vi "流程文件XML解析.vi"(10 "添加的路径":path, 11 "参数簇":cluster{"启动参数":u16, "启动模式":u16, "量程":u16}={"启动参数"=1, "启动模式"=0, "量程"=0} {"量程" items=["低量程", "高量程"]; "启动参数" items=["CODMn"=21, "总磷"=1, "总氮"=2, "氨氮"=3]; "启动模式" items=["", "水样测量", "标样核查", "零点核查", "跨度核查", "空白测试", "平行样测试", "加标回收", "填充管路", "清洗管路", "清洗反应杯"]}) -> (3 "数组":T1(array[cluster]))   [LabVIEW 2016, in "挥发酚.lvlib"]
uses:
  <vilib>/xml/Load XML File.vi
  <vilib>/xml/Close Reference(Node).vi
  <resource>/objmgr/DOMUserDefRef.rc
  <vilib>/xml/NI_XML.lvlib
panel:
  out "大小":i32
  out "XML字符串":string="<?xml version=\"1.0\" encoding=\"ISO-8859-1\"?>\n<bookstore>\n<book ISBN=\"978-0545128285\">\n  <title lang=\"en\">The Tales of Beedle the Bard</title>\n  <author>J. K. Rowling</author>\n  <year>2008</year>\n  <price>12.99</price>\n</book>\n<book ISBN=\"978-0316160209\">\n  <title lang=\"en\">Eclipse</title>\n  <author>Stephenie Meyer</author>\n  <year>2007</year>\n  <price>19.99</price>\n</book>\n<book ISBN=\"978-0316067928\">\n  <title lang=\"en\">Breaking Dawn</title>\n  <author>Stephenie Meyer</author>\n  <year>2008</year>\n  <price>22.99</price>\n</book>\n<book ISBN=\"978-0316017923\">\n  <title lang=\"en\">Outliers: The Story of Success</title>\n  <author>Malcolm Gladwell</author>\n  <year>2008</year>\n  <price>27.99</price>\n</book>\n<book ISBN=\"978-0596007645\">\n  <title lang=\"en\">XML in a Nutshell</title>\n  <author>Elliotte Rusty Harold</author>\n  <author>W. Scott Means</author>\n  <year>2004</year>\n  <price>39.95</price>\n</book>\n</bookstore>"
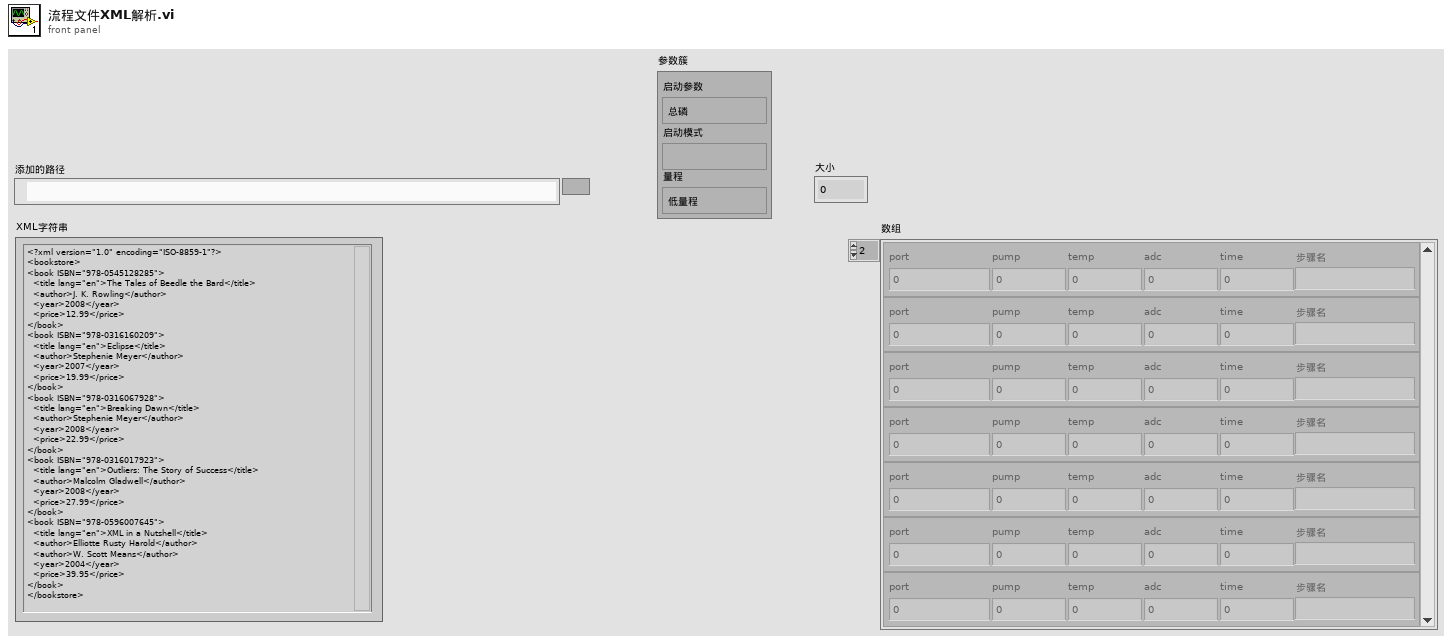
[diagram p1: front panel]
types:
  T1 = cluster{"port":u32, "pump":u16, "temp":u8, "adc":u8, "time":u16, "步骤名":string}[]
  T2 = cluster{"port":u32, "pump":u16, "temp":u8, "adc":u8, "time":u16, "步骤名":string}
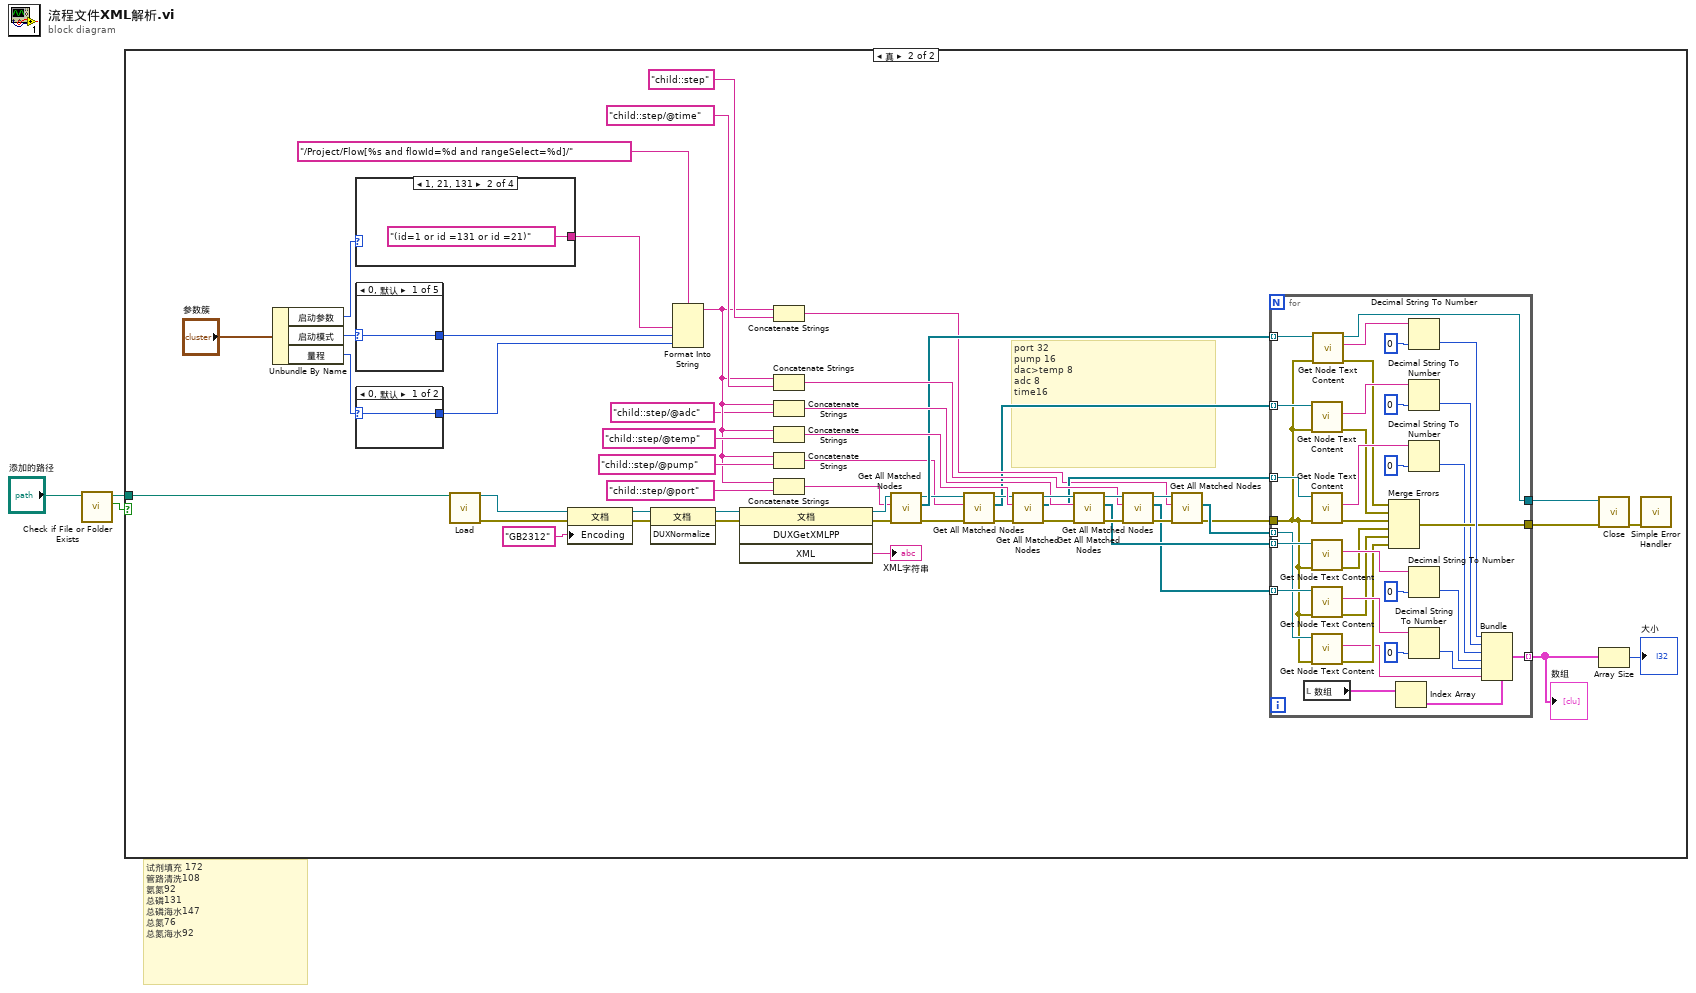
[diagram p0: block diagram]
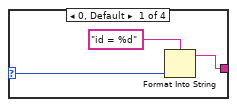
[diagram p3: hidden frame]
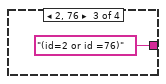
[diagram p4: hidden frame]
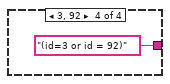
[diagram p5: hidden frame]
diagram:
  # "试剂填充 172 \n管路清洗108\n氨氮92\n总磷131\n总磷海水147\n总氮76\n总氮海水92"
  n1 = call <vilib>:"Check if File or Folder Exists.vi"("path"="添加的路径") -> ("file or folder exists?"=w1:bool, "dup path"=w2:path)  [unwired: 8 in, 1 out]
  n2 = case shown="真" w1 {
    tunnel: w2 -> [_ w40]
    frame False {
    }
    frame True {
      # "port 32\npump 16\ndac>temp 8\nadc 8\ntime16"
      n3 = Unbundle By Name("参数簇") -> ("启动参数"=w42:u16, "启动模式"=w45:u16, "量程"=w44:u16)
      n4 = case shown="1, 21, 131" w42 {
        selector: w42 -> [w93 _ _ _]
        tunnel: [w92 "(id=1 or id =131 or id =21)" ("输入 4") "(id=2 or id =76)" ("输入 4") "(id=3 or id = 92)" ("输入 4")] -> w41
        frame 0, Default {
          n5 = Format Into String(format string="id = %d" ("格式字符串"), w93) -> (resulting string=w92:string)  [unwired: 2 in, 1 out]
        }
        frame 1, 21, 131 {
        }
        frame 2, 76 {
        }
        frame 3, 92 {
        }
      }
      n6 = case shown="0, 默认" w45 {
        selector: w45 -> [w100 w101 w102 w103 w104]
        tunnel: [w100 w101 w102 w103 w104] -> w48
        frame 0, Default {
        }
        frame 1 {
        }
        frame 2 {
        }
        frame 3 {
        }
        frame 4 {
        }
      }
      n7 = case shown="0, 默认" w44 {
        selector: w44 -> [w98 w99]
        tunnel: [w98 w99] -> w47
        frame 0, Default {
        }
        frame 1 {
        }
      }
      n8 = call-poly <vilib>:"Load.vi"("path to XML document"=w40) -> ("DOM document out"=w55:refnum<k20>, "error out"=w54:errorcluster)  [unwired: 12 in, 1 out]
      n9 = property on="属性节点" class="文档"(reference=w55, error in=w54, "Encoding"="GB2312" ("文档编码")) -> (reference out=w53:refnum<k20>, error out=w52:errorcluster)
      n10 = invoke on="Invoke Node" class="文档" method="DUXNormalize"(reference=w53, error in=w52) -> (reference out=w50:refnum<k20>, error out=w51:errorcluster)  [unwired: 1 in, 1 out]
      n11 = Format Into String(format string="/Project/Flow[%s and flowId=%d and rangeSelect=%d]/" ("XPath expression"), w41, w48, w47) -> (resulting string=w8:string)  [unwired: 2 in, 1 out]
      n12 = invoke on="Invoke Node" class="文档" method="DUXGetXMLPP"(reference=w50, error in=w51) -> (reference out=w39:refnum<k20>, error out=w17:errorcluster, "XML"=→"XML字符串":string)  [unwired: 2 in, 1 out]
      n13 = Concatenate Strings(w8, "child::step" ("输入 4")) -> (w19:string)
      n14 = Concatenate Strings(w8, "child::step/@time" ("输入 4")) -> (w27:string)
      n15 = Concatenate Strings(w8, "child::step/@adc" ("输入 4")) -> (w28:string)
      n16 = Concatenate Strings(w8, "child::step/@temp" ("输入 4")) -> (w30:string)
      n17 = Concatenate Strings(w8, "child::step/@pump" ("输入 4")) -> (w7:string)
      n18 = Concatenate Strings(w8, "child::step/@port" ("输入 4")) -> (w38:string)
      n19 = call <vilib>:"Get All Matched Nodes.vi"("error in (no error)"=w17, "XPath expression"=w38, "node in"=w39) -> ("error out"=w12:errorcluster, "node result array"=w24:refnum<k20>[], "node out"=w13:refnum<k20>)  [unwired: 6 in]
      n20 = call <vilib>:"Get All Matched Nodes.vi"("error in (no error)"=w12, "XPath expression"=w7, "node in"=w13) -> ("error out"=w10:errorcluster, "node result array"=w9:refnum<k20>[], "node out"=w11:refnum<k20>)  [unwired: 6 in]
      n21 = call <vilib>:"Get All Matched Nodes.vi"("error in (no error)"=w10, "XPath expression"=w30, "node in"=w11) -> ("error out"=w36:errorcluster, "node result array"=w23:refnum<k20>[], "node out"=w35:refnum<k20>)  [unwired: 6 in]
      n22 = call <vilib>:"Get All Matched Nodes.vi"("error in (no error)"=w36, "XPath expression"=w28, "node in"=w35) -> ("error out"=w34:errorcluster, "node result array"=w22:refnum<k20>[], "node out"=w33:refnum<k20>)  [unwired: 6 in]
      n23 = call <vilib>:"Get All Matched Nodes.vi"("error in (no error)"=w34, "XPath expression"=w27, "node in"=w33) -> ("error out"=w32:errorcluster, "node result array"=w21:refnum<k20>[], "node out"=w31:refnum<k20>)  [unwired: 6 in]
      n24 = call <vilib>:"Get All Matched Nodes.vi"("error in (no error)"=w32, "XPath expression"=w19, "node in"=w31) -> ("error out"=w18:errorcluster, "node result array"=w20:refnum<k20>[])  [unwired: 6 in, 1 out]
      n25 = for {
        tunnel: w24 -> [w91] mode=indexing
        tunnel: w23 -> [w90] mode=indexing
        tunnel: w22 -> [w89] mode=indexing
        tunnel: w21 -> [w88] mode=indexing
        tunnel: w20 -> [w87] mode=indexing
        tunnel: [w77] -> w6 mode=indexing
        tunnel: w18 -> [w62]
        tunnel: [w72] -> w16
        tunnel: [w71] -> w15
        tunnel: w9 -> [w63] mode=indexing
        n26 = local read "数组"() -> (w70:T1)
        n27 = call <vilib>:"Get Node Text Content.vi"("error in (no error)"=w62, "node in"=w63) -> ("error out"=w64:errorcluster, "node text"=w66:string)  [unwired: 7 in, 1 out]
        n28 = call <vilib>:"Get Node Text Content.vi"("error in (no error)"=w62, "node in"=w90) -> ("error out"=w76:errorcluster, "node text"=w83:string)  [unwired: 7 in, 1 out]
        n29 = call <vilib>:"Get Node Text Content.vi"("error in (no error)"=w62, "node in"=w89) -> ("error out"=w75:errorcluster, "node text"=w80:string)  [unwired: 7 in, 1 out]
        n30 = call <vilib>:"Get Node Text Content.vi"("error in (no error)"=w62, "node in"=w88) -> ("error out"=w74:errorcluster, "node text"=w79:string)  [unwired: 7 in, 1 out]
        n31 = call <vilib>:"Get Node Text Content.vi"("error in (no error)"=w62, "node in"=w87) -> ("error out"=w73:errorcluster, "node text"=w68:string)  [unwired: 7 in, 1 out]
        n32 = call <vilib>:"Get Node Text Content.vi"("error in (no error)"=w62, "node in"=w91) -> ("error out"=w65:errorcluster, "node text"=w86:string, "node out"=w71:refnum<k20>)  [unwired: 7 in]
        n33 = Merge Errors(w65, w64, w76, w75, w74, w73) -> (w72:errorcluster)
        n34 = Index Array(array=w70) -> (element=w69:T2)  [unwired: 1 in]
        n35 = Decimal String To Number(string=w86, default (0L)=u32 0 ("默认(0 I32)")) -> (number=w78:u32)  [unwired: 1 in, 1 out]
        n36 = Decimal String To Number(string=w66, default (0L)=u16 0 ("默认(0 I32)")) -> (number=w61:u16)  [unwired: 1 in, 1 out]
        n37 = Decimal String To Number(string=w83, default (0L)=u8 0 ("默认(0 I32)")) -> (number=w58:u8)  [unwired: 1 in, 1 out]
        n38 = Decimal String To Number(string=w80, default (0L)=u8 0 ("默认(0 I32)")) -> (number=w59:u8)  [unwired: 1 in, 1 out]
        n39 = Decimal String To Number(string=w79, default (0L)=u16 0 ("默认(0 I32)")) -> (number=w60:u16)  [unwired: 1 in, 1 out]
        n40 = Bundle(cluster=w69, "port"=w78, "pump"=w61, "temp"=w58, "adc"=w59, "time"=w60, "步骤名"=w68) -> (w77:T2)
      }
      "数组" <- w6
      n41 = call-poly <vilib>:"Close.vi"("error in (no error)"=w16, "node"=w15) -> ("error out"=w46:errorcluster)  [unwired: 7 out]
      n42 = Array Size(array=w6) -> (size(s)=→"大小":i32)
      n43 = call <vilib>:"Simple Error Handler.vi"("error in (no error)"=w46) -> ()  [unwired: 4 in, 5 out]
    }
  }
